vi "Manual.vi"(8 "error in (no error)":errorcluster, 10 "Manual Lamp":T1, 11 "Lamp Container in":refnum<class "Lamp Container.lvclass">) -> (0 "error out":errorcluster, 3 "Lamp Container out":refnum<class "Lamp Container.lvclass">)   [LabVIEW 2016, in "Lamp Container.lvclass"]
uses:
  Lamp Container.lvclass
  Controls/Lamps Manual.ctl
  Lamp Container.lvclass/Lamp Container.ctl
  Dummy Lamp/Dummy Lamp.lvclass
  LED/LED.lvclass
  Quartz/Quartz.lvclass
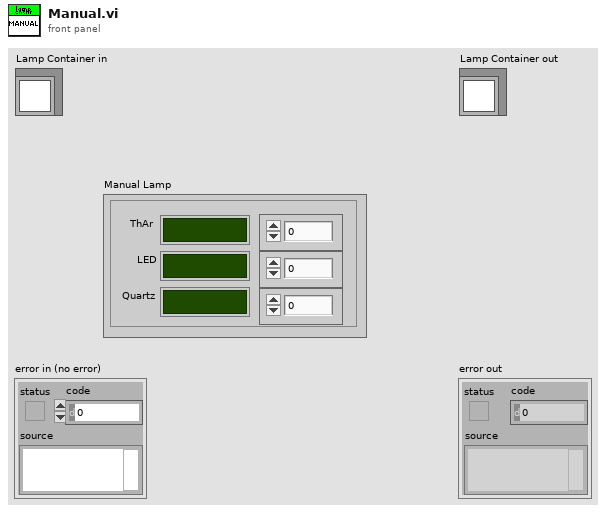
[diagram p1: front panel]
types:
  T1 = typedef "Lamps Manual.ctl" = cluster{"ThAr":bool, "Quartz":bool, "LED":bool, "ThAr Timeout":dbl, "LED Timeout":dbl, "Quartz Timeout":dbl}
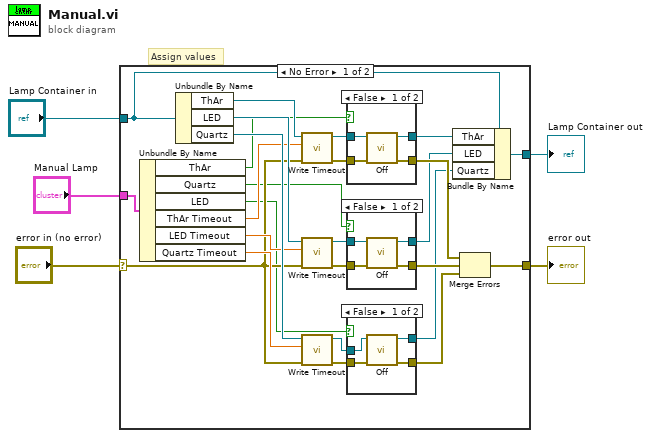
[diagram p0: block diagram]
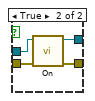
[diagram p2: hidden frame]
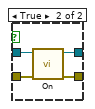
[diagram p3: hidden frame]
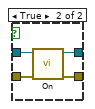
[diagram p4: hidden frame]
diagram:
  # "Assign values"
  n1 = case shown="No Error" "error in (no error)" {
    selector: "error in (no error)" -> [w22 w57]
    tunnel: [w17 w57] -> w4
    tunnel: [w31 w56] -> w2
    tunnel: "Lamp Container in" -> [w30 w56]
    tunnel: "Manual Lamp" -> [w29 _]
    frame No Error {
      n2 = Unbundle By Name(w29) -> ("ThAr"=w21:bool, "Quartz"=w15:bool, "LED"=w14:bool, "ThAr Timeout"=w25:dbl, "LED Timeout"=w24:dbl, "Quartz Timeout"=w23:dbl)
      n3 = Unbundle By Name(w30) -> ("ThAr"=w28:refnum<class "Dummy Lamp.lvclass">, "LED"=w27:refnum<class "LED.lvclass">, "Quartz"=w26:refnum<class "Quartz.lvclass">)
      n4 = call-dynamic "Write Timeout.vi"("error in (no error)"=w22, "Timeout"=w25, "Lamp in"=w28) -> ("error out"=w19:errorcluster, "Lamp out"=w20:refnum<class "Dummy Lamp.lvclass">)  [unwired: 7 in]
      n5 = call-dynamic "Write Timeout.vi"("error in (no error)"=w22, "Timeout"=w24, "Lamp in"=w27) -> ("error out"=w10:errorcluster, "Lamp out"=w12:refnum<class "LED.lvclass">)  [unwired: 7 in]
      n6 = call-dynamic "Write Timeout.vi"("error in (no error)"=w22, "Timeout"=w23, "Lamp in"=w26) -> ("error out"=w11:errorcluster, "Lamp out"=w13:refnum<class "Quartz.lvclass">)  [unwired: 7 in]
      n7 = case shown="False" w21 {
        tunnel: w20 -> [w51 w55]
        tunnel: w19 -> [w50 w53]
        tunnel: [w49 w54] -> w18
        tunnel: [w48 w52] -> w16
        frame False {
          n8 = call-dynamic "Off.vi"("error in (no error)"=w50, "Lamp in"=w51) -> ("error out"=w48:errorcluster, "Lamp out"=w49:refnum<class "Dummy Lamp.lvclass">)  [unwired: 8 in]
        }
        frame True {
          n9 = call-dynamic "On.vi"("error in (no error)"=w53, "Lamp in"=w55) -> ("error out"=w52:errorcluster, "Lamp out"=w54:refnum<class "Dummy Lamp.lvclass">)  [unwired: 8 in]
        }
      }
      n10 = case shown="False" w15 {
        tunnel: w12 -> [w43 w47]
        tunnel: w10 -> [w42 w45]
        tunnel: [w41 w46] -> w7
        tunnel: [w40 w44] -> w9
        frame False {
          n11 = call-dynamic "Off.vi"("error in (no error)"=w42, "Lamp in"=w43) -> ("error out"=w40:errorcluster, "Lamp out"=w41:refnum<class "LED.lvclass">)  [unwired: 8 in]
        }
        frame True {
          n12 = call-dynamic "On.vi"("error in (no error)"=w45, "Lamp in"=w47) -> ("error out"=w44:errorcluster, "Lamp out"=w46:refnum<class "LED.lvclass">)  [unwired: 8 in]
        }
      }
      n13 = case shown="False" w14 {
        tunnel: w13 -> [w35 w39]
        tunnel: w11 -> [w34 w37]
        tunnel: [w33 w38] -> w6
        tunnel: [w32 w36] -> w8
        frame False {
          n14 = call-dynamic "Off.vi"("error in (no error)"=w34, "Lamp in"=w35) -> ("error out"=w32:errorcluster, "Lamp out"=w33:refnum<class "Quartz.lvclass">)  [unwired: 8 in]
        }
        frame True {
          n15 = call-dynamic "On.vi"("error in (no error)"=w37, "Lamp in"=w39) -> ("error out"=w36:errorcluster, "Lamp out"=w38:refnum<class "Quartz.lvclass">)  [unwired: 8 in]
        }
      }
      n16 = Bundle By Name(cluster=w30, "ThAr"=w18, "LED"=w7, "Quartz"=w6) -> (w31:refnum<class "Lamp Container.lvclass">)
      n17 = Merge Errors(w16, w9, w8) -> (w17:errorcluster)
    }
    frame Error {
    }
  }
  "error out" <- w4
  "Lamp Container out" <- w2
